vi "CreatingSubVis.vi"() -> ()   [LabVIEW 2018]
panel:
  in  "Boolean":bool
  in  "stop":bool
  in  "Slide":dbl(slide) scale=0.0..200.0
  out "Thermometer":dbl(slide) scale=0.0..100.0
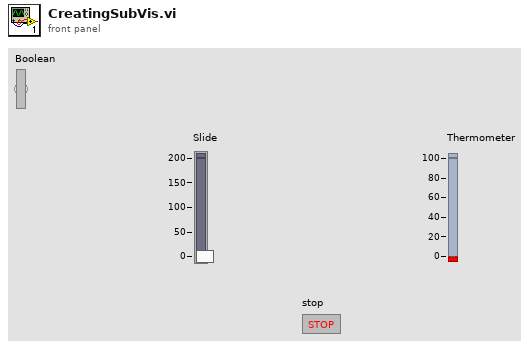
[diagram p1: front panel]
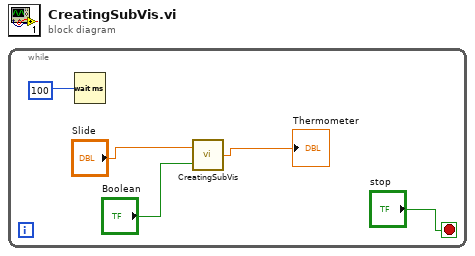
[diagram p0: block diagram]
diagram:
  n1 = while {
    stop <- "stop" stop-if-true
    n2 = Wait (ms)(milliseconds to wait=100) -> ()  [unwired: 1 out]
    n3 = call "CreatingSubVis.vi"("Boolean"="Boolean", "Slide"="Slide") -> ("Numeric"=→"Thermometer":dbl)
  }
